vi "CleanHandler.ProcConstructor.vi"(0 "i ref in":refnum<vi>, 3 "ms timeout (100)":i32=100, 5 "error in (no error)":errorcluster) -> (14 "i ref out":refnum<vi>, 17 "timed out":bool, 19 "error out":errorcluster)   [LabVIEW 2014, in "CleanHandler.lvlib"]
doc: "This method allows to do initialization (to serve as a constructor for attributes). It is necessary, since the BaseProcess.i attribute is not initialized when the ClassName.constructor is executed."
uses:
  CleanHandler.lvlib
  CSCore/CSSystem/CoreDefs/CoreDefs.error_type.ctl
  CSCore/CSSystem/CoreLib/CoreLib.string 2 byte array.vi
  CSCore/BaseProcess/BaseProcess.lvlib
  CSCore/CSSystem/CoreLib/CoreLib.lvlib
  CSCore/CSSystem/CSSystemLib/CSSystemLib.lvlib
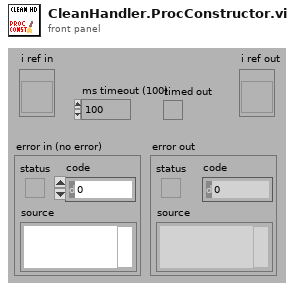
[diagram p1: front panel]
types:
  T1 = typedef "CoreDefs.error_type.ctl" = enum16{"no error", "can't load process", "can't unload process", "process does not exist", "can't install process", "can't remove process", "unknown function", "time out", "can't execute function", "duplicate queue name", "super not found", "caller queue invalid", "can't ping process", "unknown error", "VISA Error", "VISA timeout", "GPIB timeout", "GPIB error", "communication error", "data type mismatch", "can't read data from OPC server", "can't write data to OPC server", "OET error", "function not implemented", "process already exists", "invalid Shared Variable name", "error writing Shared Variable", "error reading Shared Variable", "invalid client name", "corrupt database", "unknown class", "call not authorized", "parameter out of range", "OET timeout: can't get data to modify", "invalid queue name", "requested operation incompatible with current state", "event undefined", "event disabled", "state undefined", "caller is not a friend", "EventBuilder: bad eventID", "EventBuilder: no DAQ devices", "a thread must not stop itself", "UNUSED ELEMENT4", "DiscArchiver: eventData incomplete", "DiscArchiver: eventData does not belong to run", "DiscArchiver: can't open file", "DiscArchiver: can't write to file", "DiscArchiver: available disc space low", "can't acquire semaphore", "error reading data from database", "notifier object is not existing", "can't register process", "can't unregister process", "illegal event type", "object disabled", "object already exists", "can't change state", "Instrument not found", "no connection to remote node", "invalid reference", "N/A", "UNUSED ELEMENT 1", "element not found", "illegal TCP/IP connection detected", "object does not exist", "invalid access ID", "unknown CS system", "invalid privilige", "unsupported data type", "unsupported server type", "IO server already exists", "Shared Variable already exists"}
  T2 = enum16{"simple", "synchronous", "asynchronous", "notification"}
  T3 = typedef "CoreDefs.rawDataType.ctl" = i8[]
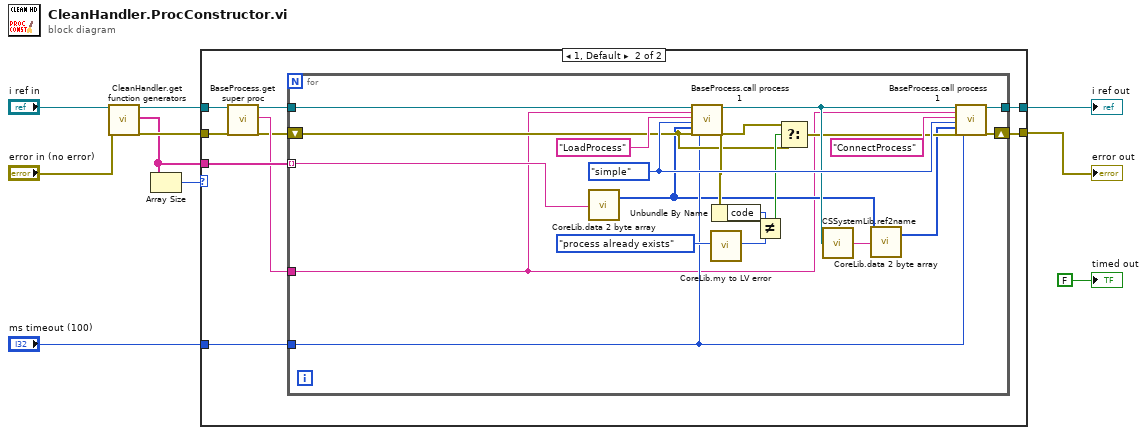
[diagram p0: block diagram]
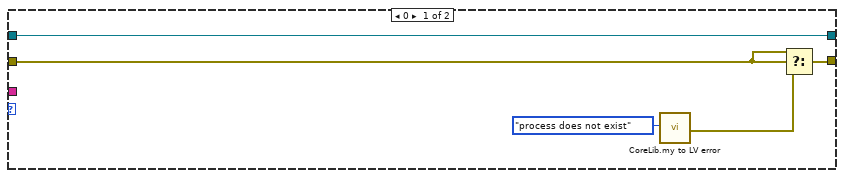
[diagram p2: hidden frame]
diagram:
  n1 = call "CleanHandler.get function generators.vi"("i ref in"="i ref in", "error in (no error)"="error in (no error)") -> ("i ref out"=w7:refnum<vi>, "function generators"=w5:string[], "error out"=w6:errorcluster)  [unwired: 14 in, 1 out]
  n2 = Array Size(array=w5) -> (size(s)=w8:i32)
  n3 = case shown="1, Default" w8 {
    tunnel: w7 -> [w15 w24]
    tunnel: w6 -> [w13 w23]
    tunnel: w5 -> [_ w21]
    tunnel: "ms timeout (100)" -> [_ w19]
    tunnel: [w14 w16] -> w3
    tunnel: [w15 w18] -> w2
    frame 0 {
      n4 = call "CoreLib.my to LV error.vi"("ErrorTypes"=CoreDefs.error_type."process does not exist") -> ("myErrorCluster"=w12:errorcluster)  [unwired: 17 in, 1 out]
      n5 = Select(t=w13, s=w13, f=w12) -> (s? t:f=w14:errorcluster)
    }
    frame 1, Default {
      n6 = call "BaseProcess.get super proc.vi"("i ref in"=w24, "error in (no error)"=w23) -> ("i ref out"=w22:refnum<vi>, "SuperProc"=w20:string, "error out"=w17:errorcluster)  [unwired: 15 in]
      n7 = for {
        tunnel: w22 -> [w44]
        tunnel: w21 -> [w29] mode=indexing
        tunnel: w20 -> [w25]
        tunnel: w19 -> [w30]
        tunnel: [w33] -> w18
        shift-right: [w31] -> w16
        shift-left: w17 -> [w32]
        w42 = T2."simple" ("CallType")
        n8 = call-poly "CoreLib.data 2 byte array.vi"("string"=w29) -> ("byteArray out"=w26:T3)  [unwired: 18 in]
        n9 = call "BaseProcess.call process 1.vi"("i ref in"=w44, "Object"=w25, "Selector"="LoadProcess", "CallType"=w42, "Data"=w26, "error in (no error)"=w32, "timeout (ms)"=w30) -> ("i ref out"=w41:refnum<vi>, "error out"=w40:errorcluster)  [unwired: 10 in, 1 out]
        n10 = call "CoreLib.my to LV error.vi"("ErrorTypes"=CoreDefs.error_type."process already exists") -> ("LV error code"=w38:i32)  [unwired: 17 in, 1 out]
        n11 = Unbundle By Name(w40) -> ("code"=w39:i32)
        n12 = Not Equal?(x=w39, y=w38) -> (x != y?=w35:bool)
        n13 = Select(t=w40, s=w35, f=w32) -> (s? t:f=w34:errorcluster)
        n14 = call "CSSystemLib.ref2name.vi"("obj refnum"=w41) -> ("name"=w28:string)
        n15 = call-poly "CoreLib.data 2 byte array.vi"("byteArray"=w26, "string"=w28) -> ("byteArray out"=w27:T3)  [unwired: 17 in]
        n16 = call "BaseProcess.call process 1.vi"("i ref in"=w41, "Object"=w25, "Selector"="ConnectProcess", "CallType"=w42, "Data"=w27, "error in (no error)"=w34, "timeout (ms)"=w30) -> ("i ref out"=w33:refnum<vi>, "error out"=w31:errorcluster)  [unwired: 10 in, 1 out]
      }
    }
  }
  "error out" <- w3
  "i ref out" <- w2
  "timed out" <- FALSE ("timed out")
